vi "Session ReLoad.vi"(8 "error in (no error)":errorcluster, 11 "ONNX Class in":refnum<class "ONNX Class.lvclass">) -> (0 "error out":errorcluster, 3 "ONNX Class out":refnum<class "ONNX Class.lvclass">)   [LabVIEW 2017, in "ONNX Class Library.lvlib" / "ONNX Class.lvclass"]
uses:
  ONNX Class.lvclass
  ONNX Class.lvclass/ONNX Class.ctl
  ONNX Class Library.lvlib
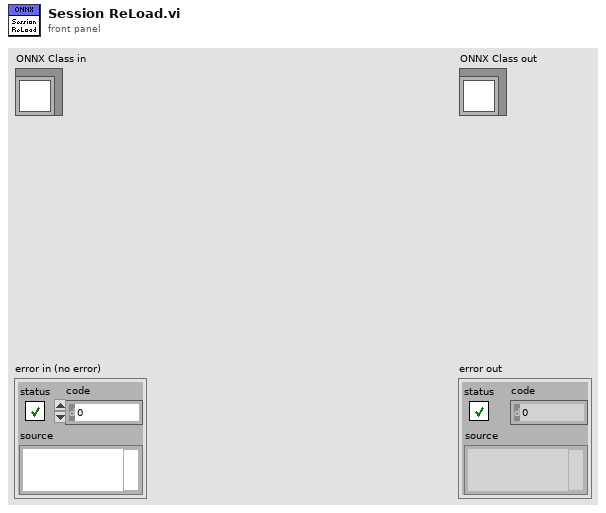
[diagram p1: front panel]
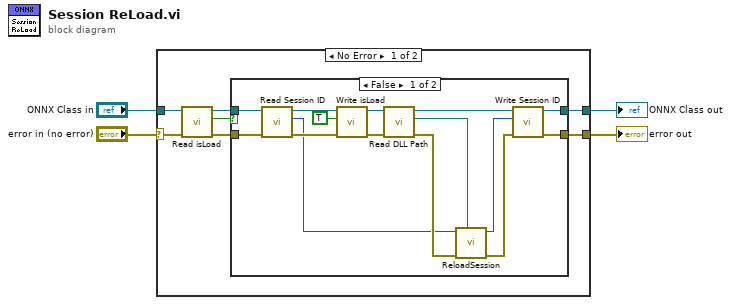
[diagram p0: block diagram]
diagram:
  n1 = case shown="No Error" "error in (no error)" {
    selector: "error in (no error)" -> [w5 w30]
    tunnel: [w7 w30] -> w2
    tunnel: [w10 w29] -> w3
    tunnel: "ONNX Class in" -> [w6 w29]
    frame No Error {
      n2 = call-dynamic "Read isLoad.vi"("error in (no error)"=w5, "ONNX Class in"=w6) -> ("error out"=w8:errorcluster, "isLoad"=w9:bool, "ONNX Class out"=w11:refnum<class "ONNX Class.lvclass">)  [unwired: 7 in]
      n3 = case shown="False" w9 {
        tunnel: [w20 w27] -> w7
        tunnel: w11 -> [w25 w28]
        tunnel: [w21 w28] -> w10
        tunnel: w8 -> [w23 w27]
        frame False {
          n4 = call-dynamic "Read Session ID.vi"("error in (no error)"=w23, "ONNX Class in"=w25) -> ("error out"=w22:errorcluster, "Session ID"=w13:i32, "ONNX Class out"=w24:refnum<class "ONNX Class.lvclass">)  [unwired: 7 in]
          n5 = call-dynamic "Write isLoad.vi"("error in (no error)"=w22, "isLoad"=TRUE, "ONNX Class in"=w24) -> ("error out"=w16:errorcluster, "ONNX Class out"=w17:refnum<class "ONNX Class.lvclass">)  [unwired: 7 in]
          n6 = call-dynamic "Read DLL Path.vi"("error in (no error)"=w16, "ONNX Class in"=w17) -> ("error out"=w15:errorcluster, "DLL Path"=w12:path, "ONNX Class out"=w14:refnum<class "ONNX Class.lvclass">)  [unwired: 7 in]
          n7 = call "ReloadSession.vi"("DLL path"=w12, "error in (no error)"=w15, "session id in"=w13) -> ("error out"=w19:errorcluster, "session id out"=w18:i32)  [unwired: 7 in]
          n8 = call-dynamic "Write Session ID.vi"("error in (no error)"=w19, "Session ID"=w18, "ONNX Class in"=w14) -> ("error out"=w20:errorcluster, "ONNX Class out"=w21:refnum<class "ONNX Class.lvclass">)  [unwired: 7 in]
        }
        frame True {
        }
      }
    }
    frame Error {
    }
  }
  "error out" <- w2
  "ONNX Class out" <- w3
